vi "Log_Reference_Velocity.vi"(1 "Measured Velocity":dbl) -> ()   [LabVIEW 2010]
uses:
  Controls/Server_Comms.ctl
  Controls/Post_Process.ctl
  Globals/Meas_global.vi
  Globals/Preference_global.vi
  Globals/Constants_global.vi
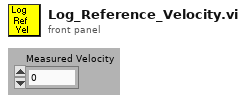
[diagram p1: front panel]
types:
  T1 = typedef "Post_Process.ctl" = enum16{"Take New Data", "Post Process Raw Data File"}
  T2 = typedef "Server_Comms.ctl" = enum16{"Server Link Healthy", "Do Not Link To Server"}
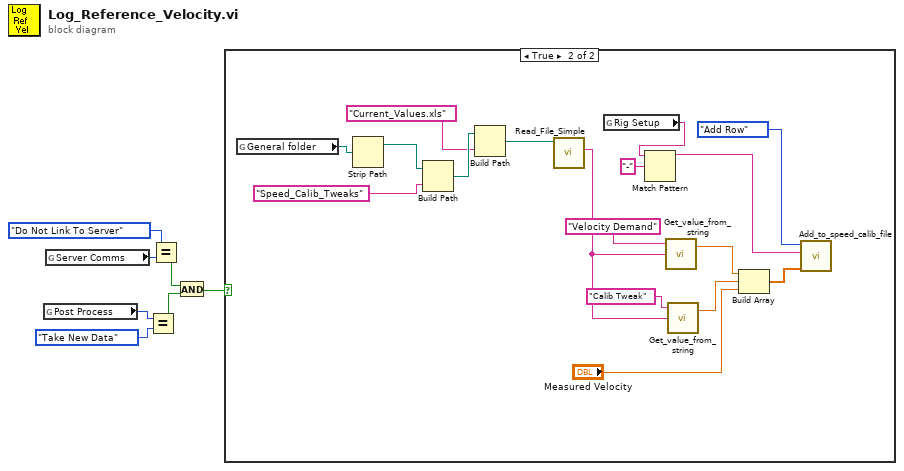
[diagram p0: block diagram]
diagram:
  n1 = global read "Meas_global.vi" "Post Process"() -> (w6:T1)
  n2 = global read "Preference_global.vi" "Server Comms"() -> (w5:T2)
  n3 = Equal?(x=w6, y=Post_Process."Take New Data" ("Post Process")) -> (x = y?=w3:bool)
  n4 = Equal?(x=Server_Comms."Do Not Link To Server" ("Server Comms"), y=w5) -> (x = y?=w2:bool)
  n5 = And(x=w2, y=w3) -> (x .and. y?=w1:bool)
  n6 = case shown="True" w1 {
    frame False {
    }
    frame True {
      n7 = global read "Constants_global.vi" "General folder"() -> (w24:path)
      n8 = Strip Path(path=w24) -> (stripped path=w23:path)  [unwired: 1 out]
      n9 = Build Path(base path=w23, name or relative path="Speed_Calib_Tweaks" ("Input Element")) -> (appended path=w21:path)
      n10 = Build Path(base path=w21, name or relative path="Current_Values.xls") -> (appended path=w19:path)
      n11 = call "Read_File_Simple.vi"("Filename"=w19) -> ("string"=w18:string)  [unwired: 2 in, 7 out]
      n12 = global read "Preference_global.vi" "Rig Setup"() -> (w10:string)
      n13 = Match Pattern(string=w10, regular expression="-") -> (before substring=w8:string)  [unwired: 4 out]
      n14 = call "Get_value_from_string.vi"("Input string"=w18, "Variable name"="Velocity Demand") -> ("Value"=w15:dbl)  [unwired: 1 in, 1 out]
      n15 = call "Get_value_from_string.vi"("Input string"=w18, "Variable name"="Calib Tweak") -> ("Value"=w14:dbl)  [unwired: 1 in, 1 out]
      n16 = Build Array(w15, w14, "Measured Velocity") -> (w12:dbl[])
      n17 = call "Add_to_speed_calib_file.vi"("New Row"=w12, "Rig Name"=w8, "Mode"=enum16{"Add Row", "Get Error Value"}."Add Row") -> ()  [unwired: 3 in, 2 out]
    }
  }
